vi "10.Pushbutton_0.vi"() -> ()   [LabVIEW 2015]
uses:
  <vilib>/myRIO/Instrument Drivers/Onboard IO/DIO/vis/Read.vi
  <vilib>/myRIO/Common/Instrument Driver Framework/myRIO v1.0/UART/vis/myRIO v1.0 Close UART.vi
  <vilib>/myRIO/Instrument Drivers/Onboard IO/DIO/vis/Smart Open.vi
  <vilib>/Utility/error.llb/Error Cluster From Error Code.vi
  <vilib>/myRIO/Common/Instrument Driver Framework/myRIO v1.0/DIO/vis/myRIO v1.0 Read DIO.vi
  <vilib>/myRIO/Common/Instrument Driver Framework/Utilities/vis/FPGA Ref Manager.vi
  <vilib>/myRIO/Common/Instrument Driver Framework/myRIO v1.0/myRIO v1.0 Reset FPGA.vi
  <vilib>/myRIO/Common/Instrument Driver Framework/myRIO v1.0/IRQ/vis/myRIO v1.0 IRQ Info FGV.vi
  <vilib>/myRIO/Common/Instrument Driver Framework/myRIO v1.0/IRQ/vis/myRIO v1.0 Timer IRQ Info FGV.vi
  <vilib>/myRIO/Common/Instrument Driver Framework/myRIO v1.0/IRQ/vis/myRIO v1.0 ISR Agent.vi
  <vilib>/myRIO/Instrument Drivers/Utilities/Utilities.lvlib
panel:
  in  "Tab Control":enum32{"Page 1", "Page 2"}(tab)
  out "LED":bool
  in  "?":bool
  out "Counter":i32
  # "Pushbutton"
  # "Pardeep kumar"
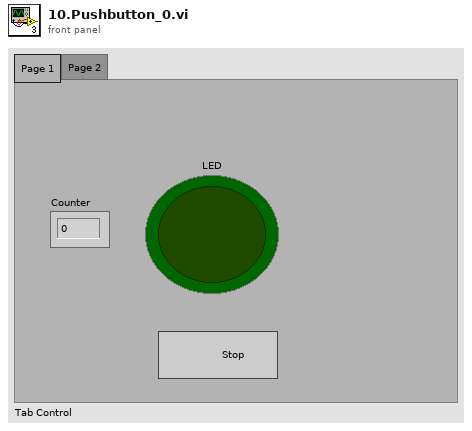
[diagram p1: front panel]
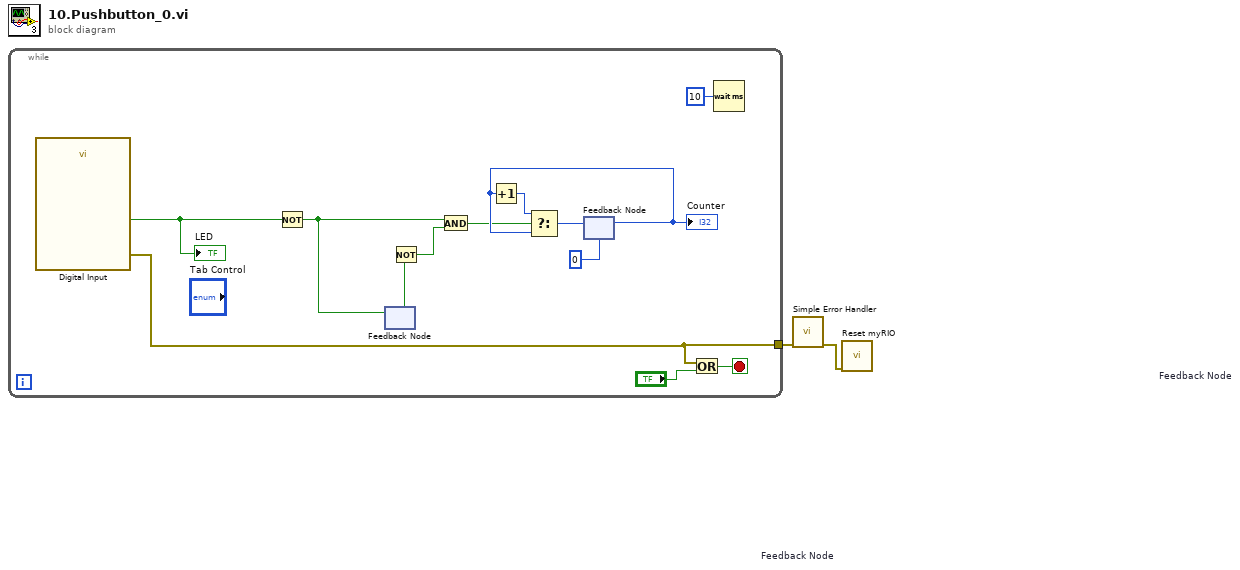
[diagram p0: block diagram]
diagram:
  n1 = while {
    tunnel: [w12] -> w2
    stop <- w15 stop-if-true
    n2 = call "Digital Input"() -> ("B/DIO0 (Pin 11)"=w6:bool, "error out"=w12:errorcluster)  [unwired: 24 in, 2 out]
    "LED" <- w6
    n3 = Not(x=w6) -> (.not. x?=w4:bool)
    n4 = feedback-in #1(w4) -> ()
    n5 = feedback #1 "Feedback Node"() -> (w3:bool)  [unwired: 1 in]
    n6 = Not(x=w3) -> (.not. x?=w7:bool)
    n7 = And(x=w4, y=w7) -> (x .and. y?=w5:bool)
    n8 = feedback #2 "Feedback Node"(0) -> (w8:i32)
    "Counter" <- w8
    n9 = Increment(x=w8) -> (x+1=w10:i32)
    n10 = Select(t=w10, s=w5, f=w8) -> (s? t:f=w9:i32)
    n11 = feedback-in #2(w9) -> ()
    n12 = Or(x=w12, y="?") -> (x .or. y?=w15:bool)
    n13 = Wait (ms)(milliseconds to wait=u32 10) -> ()  [unwired: 1 out]
  }
  n14 = call <vilib>:"Simple Error Handler.vi"("error in (no error)"=w2) -> ("error out"=w1:errorcluster)  [unwired: 4 in, 4 out]
  n15 = call <vilib>:"Reset myRIO.vi"("error in (no error)"=w1) -> ()  [unwired: 10 in, 1 out]
